vi "Save VI with XML Heaps.vi"(8 "error in (no error)":errorcluster, 10 "VI Path (temporary file)":path=path "", 11 "VI Refnum In":refnum<vi>) -> (0 "error out":errorcluster, 2 "VI Path out":path, 3 "VI Refnum Out":refnum<vi>)   [LabVIEW 2015]
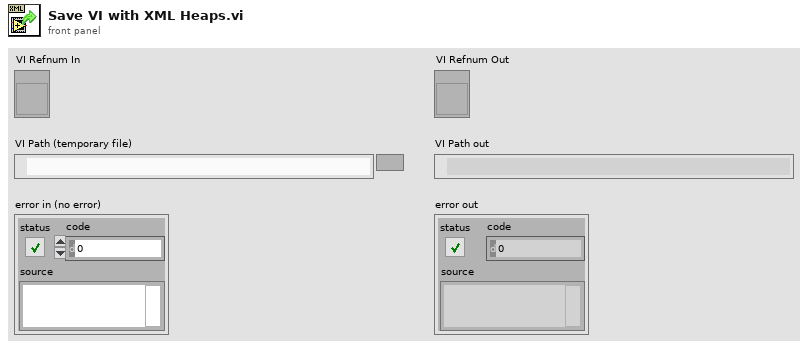
[diagram p1: front panel]
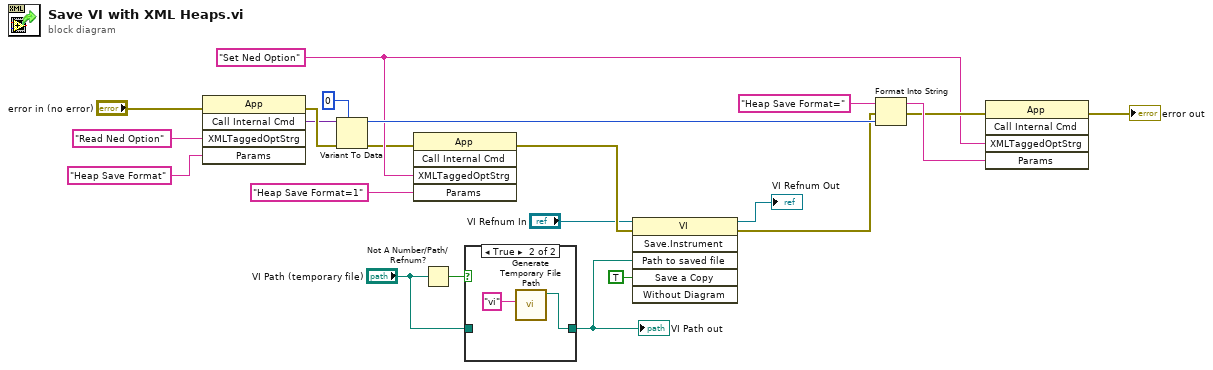
[diagram p0: block diagram]
diagram:
  w13 = "Set Ned Option" ("Command Name")
  n1 = invoke class="App" method="Call Internal Cmd"(error in="error in (no error)", "XMLTaggedOptStrg"="Read Ned Option" ("Command Name"), "Params"="Heap Save Format") -> (error out=w22:errorcluster, "CallInternalCmd"=w19:variant)  [unwired: 2 in, 3 out]
  n2 = Variant To Data(error in=w22, type=0, Variant=w19) -> (data=w16:i32, error out=w12:errorcluster)
  n3 = invoke class="App" method="Call Internal Cmd"(error in=w12, "XMLTaggedOptStrg"=w13, "Params"="Heap Save Format=1") -> (error out=w10:errorcluster)  [unwired: 2 in, 4 out]
  n4 = Not A Number/Path/Refnum?(number/path/refnum="VI Path (temporary file)") -> (NaN/Path/Refnum?=w4:bool)
  n5 = case shown="True" w4 {
    tunnel: [w23 w25] -> w2
    tunnel: "VI Path (temporary file)" -> [w23 _]
    frame False {
    }
    frame True {
      n6 = call <vilib>:"Generate Temporary File Path.vi"("Temporary File Extension (tmp)"="vi") -> ("Unique Temporary File Path"=w25:path)  [unwired: 9 in, 1 out]
    }
  }
  "VI Path out" <- w2
  n7 = invoke class="VI" method="Save.Instrument"(reference="VI Refnum In", error in=w10, "Path to saved file"=w2, "Save a Copy"=TRUE) -> (reference out=→"VI Refnum Out":refnum<vi>, error out=w9:errorcluster)  [unwired: 2 in, 4 out]
  n8 = Format Into String(initial string="Heap Save Format=", error in=w9, w16) -> (resulting string=w15:string, error out=w14:errorcluster)  [unwired: 1 in]
  n9 = invoke class="App" method="Call Internal Cmd"(error in=w14, "XMLTaggedOptStrg"=w13, "Params"=w15) -> (error out=→"error out":errorcluster)  [unwired: 2 in, 4 out]
